vi "TX DO Pulse Done.vi"(8 "error in (no error)":errorcluster, 9 "Success?":bool, 10 "Port Number":u8, 11 "DUT Sample in":refnum<class "DUT Sample.lvclass">) -> (0 "error out":errorcluster, 3 "DUT Sample out":refnum<class "DUT Sample.lvclass">)   [LabVIEW 2023, in "DUT Sample.lvclass"]
uses:
  DUT Sample.lvclass
  DUT Sample.lvclass/DUT Sample.ctl
  <vilib>/xnet/xnet.llb/XNET Write (Signal Single-point).vi
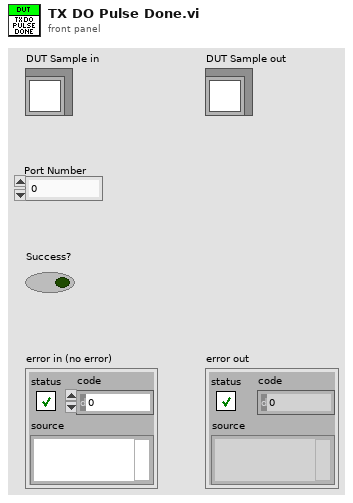
[diagram p1: front panel]
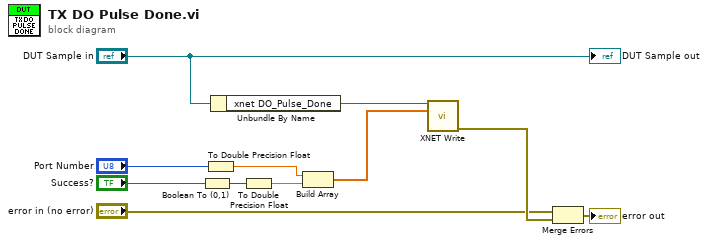
[diagram p0: block diagram]
diagram:
  n1 = Boolean To (0,1)(Boolean="Success?") -> (0, 1=w7:i16)
  n2 = To Double Precision Float(number="Port Number") -> (double precision float=w5:dbl)
  n3 = Unbundle By Name("DUT Sample in") -> ("xnet DO_Pulse_Done"=w8:refnum<k21>)
  n4 = To Double Precision Float(number=w7) -> (double precision float=w6:dbl)
  n5 = Build Array(w5, w6) -> (w4:dbl[])
  n6 = call-poly <vilib>:"XNET Write.vi"("session in"=w8, "data"=w4) -> ("error out"=w2:errorcluster)  [unwired: 12 in, 1 out]
  n7 = Merge Errors("error in (no error)", w2) -> (→"error out":errorcluster)
  "DUT Sample out" <- "DUT Sample in"
